vi "wd_append (WFM).vi"(6 "data type":T7, 7 "Waveform":waveform(dbl), 8 "error in (no error)":errorcluster, 9 "channel index":u32, 11 "meta in":T1={"TargetFile"=path "", "StreamMode"=enum."File", "Append?"=FALSE, "ChunkSize"=0, "TimeColumnMode"=enum."Empty", "TimestampFormat"="", "AbsoluteTime?"=FALSE, "FileAttribute "={"Creator"="", "Title"="", "SheetName"=""}, "Column"=[], "FileRef"=refnum, "MemoryRef"=[], "RecordInfo"=[], " ChannelPreviousInfo"=[], "ChannelFirstRecord"=[], "PredefinedFormattedValueLength"=20, "DiskTemplate"={"XMLRef"=[refnum, refnum, refnum, refnum, refnum, refnum], "ZipPath"=path "", "MetaFile"={"Ref"=refnum, "NextRow"=0, "NextPosition"=0, "Block"=[]}, "TempFolder"=path ""}}) -> (0 "error out":errorcluster, 3 "meta out":T1={"TargetFile"=path "", "StreamMode"=enum."File", "Append?"=FALSE, "ChunkSize"=0, "TimeColumnMode"=enum."Empty", "TimestampFormat"="", "AbsoluteTime?"=FALSE, "FileAttribute "={"Creator"="", "Title"="", "SheetName"=""}, "Column"=[], "FileRef"=refnum, "MemoryRef"=[], "RecordInfo"=[], " ChannelPreviousInfo"=[], "ChannelFirstRecord"=[], "PredefinedFormattedValueLength"=20, "DiskTemplate"={"XMLRef"=[refnum, refnum, refnum, refnum, refnum, refnum], "ZipPath"=path "", "MetaFile"={"Ref"=refnum, "NextRow"=0, "NextPosition"=0, "Block"=[]}, "TempFolder"=path ""}})   [LabVIEW 2020, in "NI_ExcelFile.lvlib"]
uses:
  <vilib>/express/express shared/NI_ExcelFile/NI_ExcelFile.lvlib
  <vilib>/express/express shared/NI_ExcelFile/Ctrls/DataType.ctl
  <vilib>/express/express shared/NI_ExcelFile/Ctrls/MainData.ctl
  <vilib>/express/express shared/NI_ExcelFile/Ctrls/StreamMode.ctl
  <vilib>/express/express shared/NI_ExcelFile/Ctrls/TimeColumnMode.ctl
  <vilib>/express/express shared/NI_ExcelFile/Ctrls/FileAttribute.ctl
  <vilib>/express/express shared/NI_ExcelFile/Ctrls/Columns.ctl
  <vilib>/express/express shared/NI_ExcelFile/Ctrls/ColumnInfo.ctl
  <vilib>/express/express shared/NI_ExcelFile/Ctrls/wd_recordInfo.ctl
  <vilib>/express/express shared/NI_ExcelFile/Ctrls/disk_TemplateFile.ctl
  <vilib>/express/express shared/NI_ExcelFile/Ctrls/meta_file.ctl
  <vilib>/express/express shared/NI_ExcelFile/Ctrls/meta_Block.ctl
  <vilib>/express/express shared/NI_ExcelFile/Ctrls/meta_BlockType.ctl
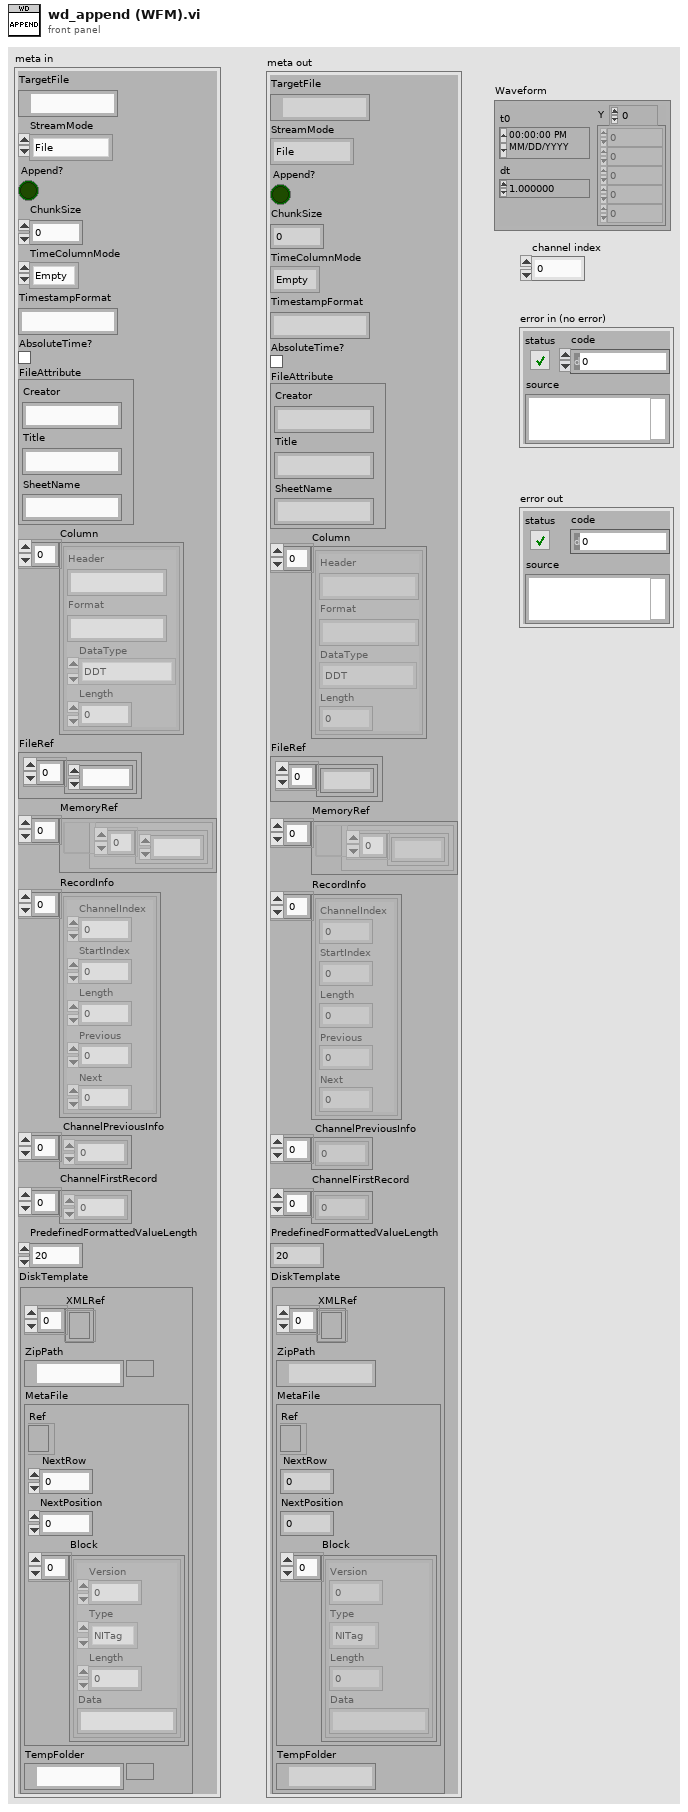
[diagram p1: front panel]
types:
  T1 = typedef "NI_ExcelFile.lvlib/MainData.ctl" = cluster{"TargetFile":path, "StreamMode":T2, "Append?":bool, "ChunkSize":u64, "TimeColumnMode":T3, "TimestampFormat":string, "AbsoluteTime?":bool, "FileAttribute ":T4, "Column":T5, "FileRef":refnum<k1>, "MemoryRef":refnum<data-value>[], "RecordInfo":T8[], " ChannelPreviousInfo":u32[], "ChannelFirstRecord":u32[], "PredefinedFormattedValueLength":i64, "DiskTemplate":T9}
  T2 = typedef "NI_ExcelFile.lvlib/StreamMode.ctl" = enum16{"File", "Memory"}
  T3 = typedef "NI_ExcelFile.lvlib/TimeColumnMode.ctl" = enum16{"Empty", "OnePerCh", "One"}
  T4 = typedef "NI_ExcelFile.lvlib/FileAttribute.ctl" = cluster{"Creator":string, "Title":string, "SheetName":string}
  T5 = typedef "NI_ExcelFile.lvlib/Columns.ctl" = T6[]
  T6 = typedef "NI_ExcelFile.lvlib/ColumnInfo.ctl" = cluster{"Header":string, "Format":string, "DataType":T7, "Length":u64}
  T7 = typedef "NI_ExcelFile.lvlib/DataType.ctl" = enum16{"DDT", "WFM", "Array of STR", "Array of DBL", "Array of I8", "Array of I16", "Array of I32", "Array of I64", "Array of SGL", "Array of U8", "Array of U16", "Array of U32", "Array of U64", "Array of Time"}
  T8 = typedef "NI_ExcelFile.lvlib/wd_recordInfo.ctl" = cluster{"ChannelIndex":u32, "StartIndex":u64, "Length":u64, "Previous":i32, "Next":i32}
  T9 = typedef "NI_ExcelFile.lvlib/disk_TemplateFile.ctl" = cluster{"XMLRef":refnum<file>[], "ZipPath":path, "MetaFile":T10, "TempFolder":path}
  T10 = typedef "NI_ExcelFile.lvlib/meta_file.ctl" = cluster{"Ref":refnum<file>, "NextRow":i32, "NextPosition":i64, "Block":T11[]}
  T11 = typedef "NI_ExcelFile.lvlib/meta_Block.ctl" = cluster{"Version":u16, "Type":T12, "Length":i32, "Data":string}
  T12 = typedef "NI_ExcelFile.lvlib/meta_BlockType.ctl" = enum16{"NITag", "File", "Column"}
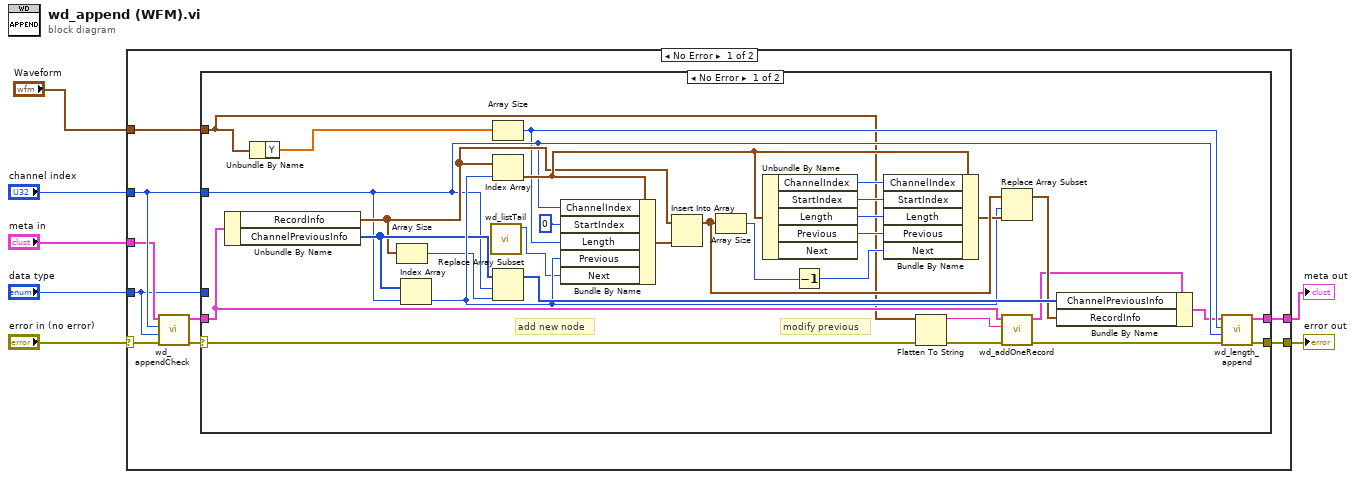
[diagram p0: block diagram]
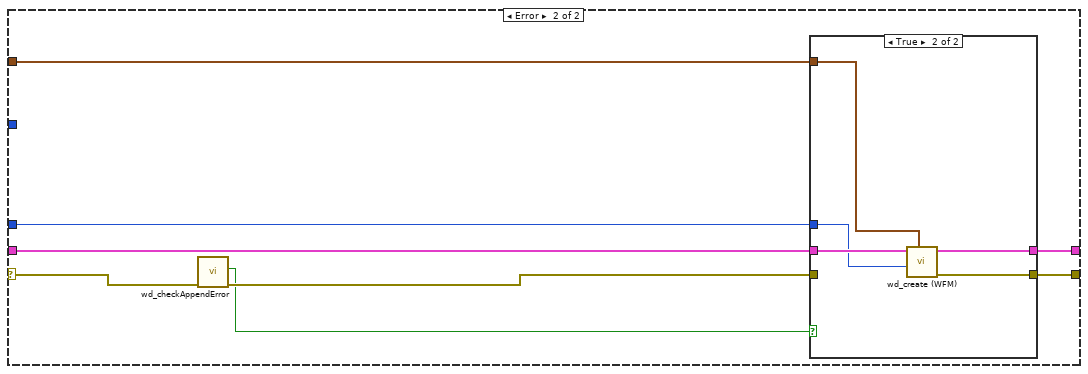
[diagram p2: hidden frame]
diagram:
  n1 = case shown="No Error" "error in (no error)" {
    selector: "error in (no error)" -> [w8 w64]
    tunnel: "data type" -> [w10 _]
    tunnel: "channel index" -> [w13 _]
    tunnel: "meta in" -> [w12 w63]
    tunnel: [w16 w63] -> w4
    tunnel: [w15 w64] -> w3
    tunnel: "Waveform" -> [w14 _]
    frame No Error {
      n2 = call <vilib>:"wd_appendCheck.vi"("error in (no error)"=w8, "DataType"=w10, "channel index (0)"=w13, "data in"=w12) -> ("error out"=w9:errorcluster, "data out"=w11:T1)  [unwired: 6 in]
      n3 = case shown="No Error" w9 {
        selector: w9 -> [w22 w50]
        tunnel: [w20 w51] -> w15
        tunnel: w11 -> [w26 w53]
        tunnel: w14 -> [w18 w55]
        tunnel: [w23 w52] -> w16
        tunnel: w13 -> [w28 _]
        tunnel: w10 -> [_ w54]
        frame No Error {
          # "modify previous"
          # "add new node"
          n4 = Unbundle By Name(w26) -> ("RecordInfo"=w31:T8[], "ChannelPreviousInfo"=w32:u32[])
          n5 = Unbundle By Name(w18) -> ("Y"=w17:dbl[])
          n6 = Array Size(array=w31) -> (size(s)=w33:i32)
          n7 = Index Array(array=w32, index=w28) -> (element=w35:u32)
          n8 = call <vilib>:"wd_listTail.vi"() -> ("list tail"=w19:i32)  [unwired: 11 in]
          n9 = Array Size(array=w17) -> (size(s)=w27:i32)
          n10 = Index Array(array=w31, index=w35) -> (element=w44:T8)
          n11 = Replace Array Subset(array=w32, new element=w33, index=w28) -> (w47:u32[])
          n12 = Bundle By Name(cluster=w44, "ChannelIndex"=w28, "StartIndex"=u64 0 ("Start Index"), "Length"=w27, "Previous"=w35, "Next"=w19) -> (w45:T8)
          n13 = Insert Into Array(array=w31, new element=w45) -> (w37:T8[])  [unwired: 1 in]
          n14 = Array Size(array=w37) -> (size(s)=w39:i32)
          n15 = Unbundle By Name(w44) -> ("ChannelIndex"=w43:u32, "StartIndex"=w42:u64, "Length"=w41:u64, "Previous"=w40:i32)  [unwired: 1 out]
          n16 = Decrement(x=w39) -> (x-1=w38:i32)
          n17 = Bundle By Name(cluster=w44, "ChannelIndex"=w43, "StartIndex"=w42, "Length"=w41, "Previous"=w40, "Next"=w38) -> (w36:T8)
          n18 = Flatten To String(anything=w18, error in (no error)=w22) -> (data string=w30:string, error out=w29:errorcluster)  [unwired: 2 in, 1 out]
          n19 = Replace Array Subset(array=w37, new element=w36, index=w35) -> (w34:T8[])
          n20 = call <vilib>:"wd_addOneRecord.vi"("error in (no error)"=w29, "data"=w30, "meta in"=w26) -> ("error out"=w21:errorcluster, "meta out"=w25:T1)  [unwired: 7 in]
          n21 = Bundle By Name(cluster=w25, "ChannelPreviousInfo"=w47, "RecordInfo"=w34) -> (w24:T1)
          n22 = call <vilib>:"wd_length_append.vi"("error in (no error)"=w21, "channel index (0)"=w28, "data size"=w27, "meta in"=w24) -> ("error out"=w20:errorcluster, "meta out"=w23:T1)  [unwired: 6 in]
        }
        frame Error {
          n23 = call <vilib>:"wd_checkAppendError.vi"("error in (no error)"=w50) -> ("error out"=w49:errorcluster, "special error?"=w48:bool)  [unwired: 9 in]
          n24 = case shown="True" w48 {
            tunnel: w53 -> [w57 w62]
            tunnel: w55 -> [_ w58]
            tunnel: w54 -> [_ w61]
            tunnel: w49 -> [w56 _]
            tunnel: [w57 w60] -> w52
            tunnel: [w56 w59] -> w51
            frame False {
            }
            frame True {
              n25 = call <vilib>:"wd_create (WFM).vi"("WFM"=w58, "data type"=w61, "meta in"=w62) -> ("error out"=w59:errorcluster, "meta out"=w60:T1)  [unwired: 7 in]
            }
          }
        }
      }
    }
    frame Error {
    }
  }
  "meta out" <- w4
  "error out" <- w3
